vi "ReadPathToPluginRequest.vi"(8 "error in (no error)":errorcluster, 11 "ModuleID":i32=-1) -> (0 "error out":errorcluster)   [LabVIEW 2014, in "PmuImpairModule.lvlib"]
uses:
  PmuImpairModule.lvlib
  clEventType.ctl
  <vilib>/Utility/error.llb/Error Cluster From Error Code.vi
  <vilib>/ErrorRing/Error Ring.xnode
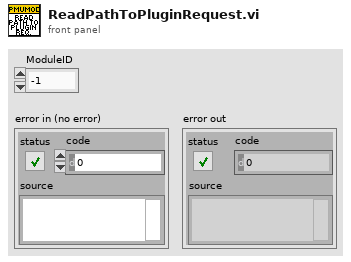
[diagram p1: front panel]
types:
  T1 = typedef "PmuImpairModule.lvlib/clRequestEvents.ctl" = cluster{"StopRequest":refnum<user-event>, "LoadPluginRequest":refnum<user-event>, "WriteImpairConfig":refnum<user-event>, "ReadImpairConfig":refnum<user-event>, "WriteImpairParams":refnum<user-event>, "ReadImpairParams":refnum<user-event>, "WriteEvtReports":refnum<user-event>, "GetImpairReports":refnum<user-event>, "ReadPathToPluginRequest":refnum<user-event>, "WriteEvtSignal":refnum<user-event>, "WriteEvtConfig":refnum<user-event>, "WriteEvtParams":refnum<user-event>, "ReadBusNumber":refnum<user-event>, "WriteBusNumber":refnum<user-event>, "ShowPanel":refnum<user-event>}
  T2 = typedef "PmuImpairModule.lvlib/clEventType.ctl" = cluster{"ModuleID":i32, "Data":variant}
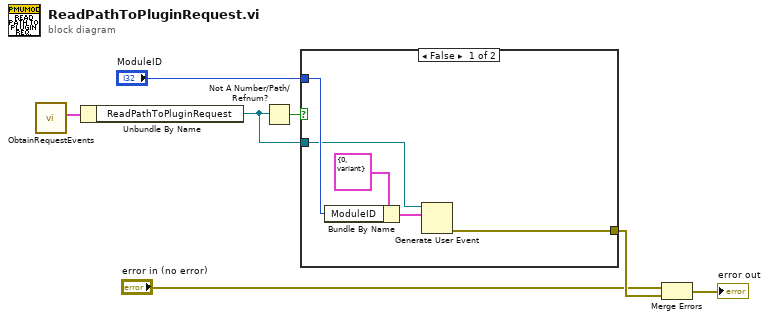
[diagram p0: block diagram]
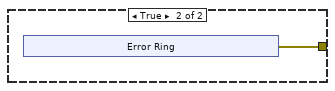
[diagram p2: hidden frame]
diagram:
  n1 = call "ObtainRequestEvents.vi"() -> ("clRequestEvents"=w7:T1)  [unwired: 10 in, 1 out]
  n2 = Unbundle By Name(w7) -> ("ReadPathToPluginRequest"=w5:refnum<user-event>)
  n3 = Not A Number/Path/Refnum?(number/path/refnum=w5) -> (NaN/Path/Refnum?=w6:bool)
  n4 = case shown="False" w6 {
    tunnel: w5 -> [w10 _]
    tunnel: "ModuleID" -> [w11 _]
    tunnel: [w8 w13] -> w2
    frame False {
      n5 = Bundle By Name(cluster=T2 {"ModuleID"=0, "Data"=variant} ("clEventType"), "ModuleID"=w11) -> (w9:T2)
      n6 = Generate User Event(user event=w10, event data cluster=w9) -> (error out=w8:errorcluster)  [unwired: 2 in, 1 out]
    }
    frame True {
      n7 = xnode "Error Ring"() -> ("error out"=w13:errorcluster)
    }
  }
  n8 = Merge Errors("error in (no error)", w2) -> (→"error out":errorcluster)
